vi "Update Stats.vi"(8 "Team":i32, 11 "Enum":T1) -> ()   [LabVIEW 2020, in "SB SubVIs.lvlib"]
uses:
  SB SubVIs.lvlib
  Type Defs/Status Enum.ctl
  Globals (private).vi
  Type Defs/SB Type Defs.lvlib
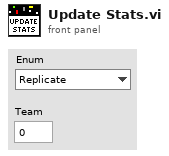
[diagram p1: front panel]
types:
  T1 = typedef "SB Type Defs.lvlib/Status Enum.ctl" = enum16{"Replicate", "Kill", "Eliminate", "Collide"}
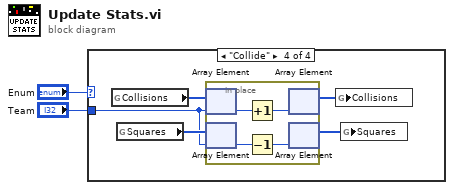
[diagram p0: block diagram]
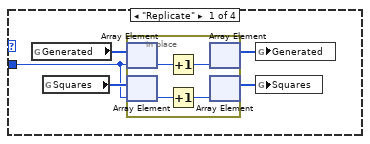
[diagram p2: hidden frame]
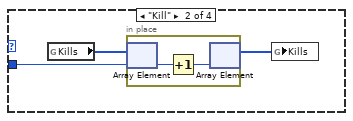
[diagram p3: hidden frame]
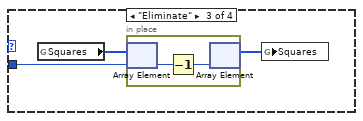
[diagram p4: hidden frame]
diagram:
  n1 = case shown="\"Collide\"" "Enum" {
    tunnel: "Team" -> [w5 w13 w18 w22]
    frame "Replicate" {
      n2 = global read "Globals (private).vi" "Generated"() -> (w7:i32[])
      n3 = global read "Globals (private).vi" "Squares"() -> (w6:i32[])
      n4 = in-place {
        n5 = in-place-array #1(w7, w5) -> (w11:i32)
        n6 = in-place-array #2(w6, w5) -> (w10:i32)
        n7 = Increment(x=w11) -> (x+1=w8:i32)
        n8 = Increment(x=w10) -> (x+1=w9:i32)
        n9 = in-place-array #1(w8) -> (w4:i32[])  [unwired: 1 out]
        n10 = in-place-array #2(w9) -> (w3:i32[])  [unwired: 1 out]
      }
      n11 = global write "Globals (private).vi" "Generated"(w4) -> ()
      n12 = global write "Globals (private).vi" "Squares"(w3) -> ()
    }
    frame "Kill" {
      n13 = global read "Globals (private).vi" "Kills"() -> (w14:i32[])
      n14 = in-place {
        n15 = in-place-array #3(w14, w13) -> (w16:i32)
        n16 = Increment(x=w16) -> (x+1=w15:i32)
        n17 = in-place-array #3(w15) -> (w12:i32[])  [unwired: 1 out]
      }
      n18 = global write "Globals (private).vi" "Kills"(w12) -> ()
    }
    frame "Eliminate" {
      n19 = global read "Globals (private).vi" "Squares"() -> (w19:i32[])
      n20 = in-place {
        n21 = in-place-array #4(w19, w18) -> (w21:i32)
        n22 = Decrement(x=w21) -> (x-1=w20:i32)
        n23 = in-place-array #4(w20) -> (w17:i32[])  [unwired: 1 out]
      }
      n24 = global write "Globals (private).vi" "Squares"(w17) -> ()
    }
    frame "Collide" {
      n25 = global read "Globals (private).vi" "Collisions"() -> (w26:i32[])
      n26 = global read "Globals (private).vi" "Squares"() -> (w23:i32[])
      n27 = in-place {
        n28 = in-place-array #5(w26, w22) -> (w30:i32)
        n29 = in-place-array #6(w23, w22) -> (w27:i32)
        n30 = Increment(x=w30) -> (x+1=w29:i32)
        n31 = Decrement(x=w27) -> (x-1=w28:i32)
        n32 = in-place-array #5(w29) -> (w25:i32[])  [unwired: 1 out]
        n33 = in-place-array #6(w28) -> (w24:i32[])  [unwired: 1 out]
      }
      n34 = global write "Globals (private).vi" "Collisions"(w25) -> ()
      n35 = global write "Globals (private).vi" "Squares"(w24) -> ()
    }
  }
